vi "S2C_VLFT10_Proc_ClearAlarms.vi"(8 "Error In":errorcluster, 11 "Alarms":string) -> (0 "Error Out":errorcluster)   [LabVIEW 2015]
uses:
  Fornax/VIs/S2C_FORNAX_Proc_Globals.vi
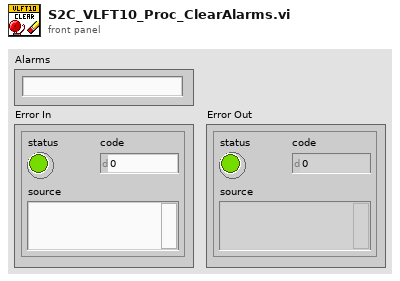
[diagram p1: front panel]
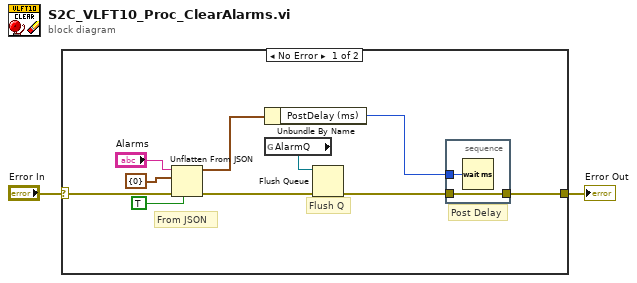
[diagram p0: block diagram]
diagram:
  n1 = case shown="No Error" "Error In" {
    selector: "Error In" -> [w12 w15]
    tunnel: [w3 w15] -> w1
    frame No Error {
      # "Post Delay"
      # "Flush Q"
      # "From JSON"
      n2 = Unflatten From JSON(JSON string="Alarms", type and defaults=cluster{"PostDelay (ms)":i32} {"PostDelay (ms)"=0}, default null elements? (F)=TRUE, error in (no error)=w12) -> (value=w5:cluster{"PostDelay (ms)":i32}, error out=w8:errorcluster)  [unwired: 3 in]
      n3 = Unbundle By Name(w5) -> ("PostDelay (ms)"=w4:i32)
      n4 = global read "S2C_FORNAX_Proc_Globals.vi" "AlarmQ"() -> (w9:refnum<queue>)
      n5 = Flush Queue(queue=w9, error in (no error)=w8) -> (error out=w6:errorcluster)  [unwired: 2 out]
      n6 = stacked-sequence {
        tunnel: w6 -> [w14]
        tunnel: [w14] -> w3
        tunnel: w4 -> [w13]
        frame #0 {
          n7 = Wait (ms)(milliseconds to wait=w13) -> ()  [unwired: 1 out]
        }
      }
    }
    frame Error {
    }
  }
  "Error Out" <- w1
